vi "Parse Start.vi"(8 "error in (no error)":errorcluster, 10 "String in":string, 11 "Request in":refnum<class "Request.lvclass">) -> (0 "error out":errorcluster, 2 "Remaining":string, 3 "Request out":refnum<class "Request.lvclass">)   [LabVIEW 2020, in "HTTP Utils.lvlib" / "Request.lvclass"]
uses:
  Request.lvclass
  Method.ctl
  Request.lvclass/Request.ctl
  HTTP Utils.lvlib
  <vilib>/IlluminatedG/lv-stream/URI/URI.lvclass
  <vilib>/IlluminatedG/lv-stream/Stream.lvlib
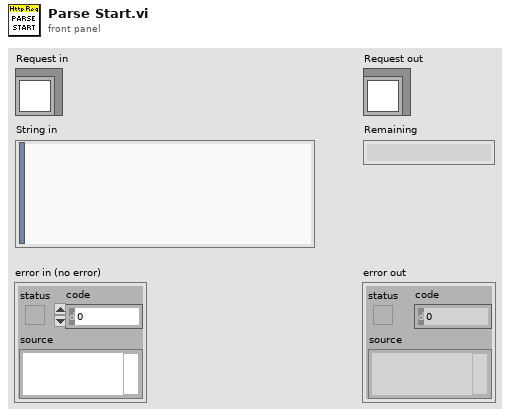
[diagram p1: front panel]
types:
  T1 = typedef "HTTP Utils.lvlib/Method.ctl" = enum16{"GET", "HEAD", "POST", "PUT", "DELETE", "CONNECT", "OPTIONS", "TRACE", "PATCH"}
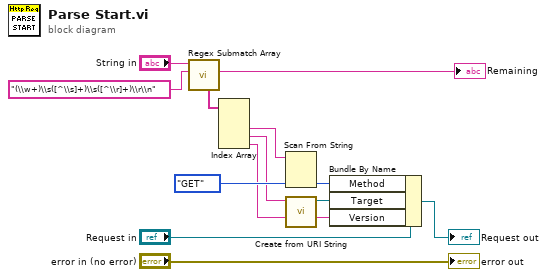
[diagram p0: block diagram]
diagram:
  n1 = call <vilib>:"Regex Submatch Array.vi"("regular expression"="(\\w+)\\s([^\\s]+)\\s([^\\r]+)\\r\\n", "string"="String in") -> ("after match"=→"Remaining":string, "matches"=w4:string[])  [unwired: 5 in, 3 out]
  n2 = Index Array(array=w4) -> (element #2=w3:string, element #3=w2:string, element #4=w1:string)  [unwired: 4 in, 1 out]
  n3 = Scan From String(input string=w3, default 1=Method."GET" ("Method")) -> (output 1=w9:T1)  [unwired: 3 in, 3 out]
  n4 = call <vilib>:"Create from URI String.vi"("URI String"=w2) -> ("URI out"=w8:refnum<class "URI.lvclass">)  [unwired: 9 in, 1 out]
  n5 = Bundle By Name(cluster="Request in", "Method"=w9, "Target"=w8, "Version"=w1) -> (→"Request out":refnum<class "Request.lvclass">)
  "error out" <- "error in (no error)"
